vi "getReadOnly.vi"(8 "error in (no error)":errorcluster, 11 "IProperty in":refnum<class "IProperty.lvclass">) -> (0 "error out":errorcluster, 2 "Read Only?":bool, 3 "IProperty out":refnum<class "IProperty.lvclass">, 5 "Read Only?":string)   [LabVIEW 2022 SP3, in "openDAQ.lvlib" / "IBaseObject.lvlib" / "IProperty.lvlib" / "IProperty.lvclass"]
uses:
  <instrlib>/openDAQ/Public/Classes/IProperty/IProperty.lvclass
  C:/Program Files (x86)/National Instruments/LabVIEW 2022/instr.lib/openDAQ/Public/Classes/IBaseObject/IBaseObject.lvclass
  <instrlib>/openDAQ/Public/Classes/IBaseObject/IBaseObject.lvclass/IBaseObject.ctl
  <instrlib>/openDAQ/Public/Classes/IBaseObject/Accessor/Read reference.vi
  <instrlib>/openDAQ/Binaries/Windows/x86/copendaq32.dll
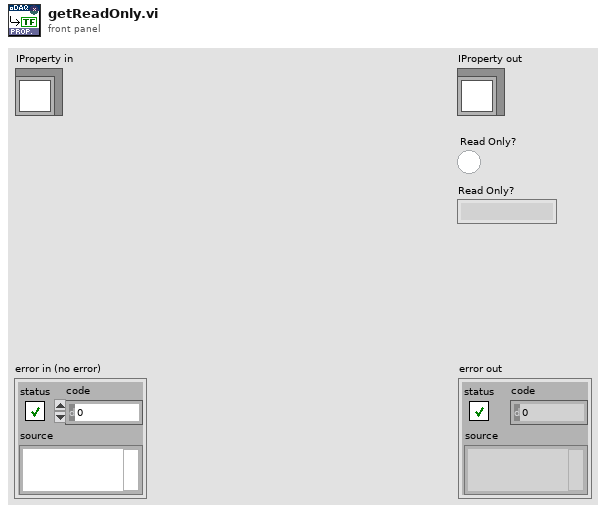
[diagram p1: front panel]
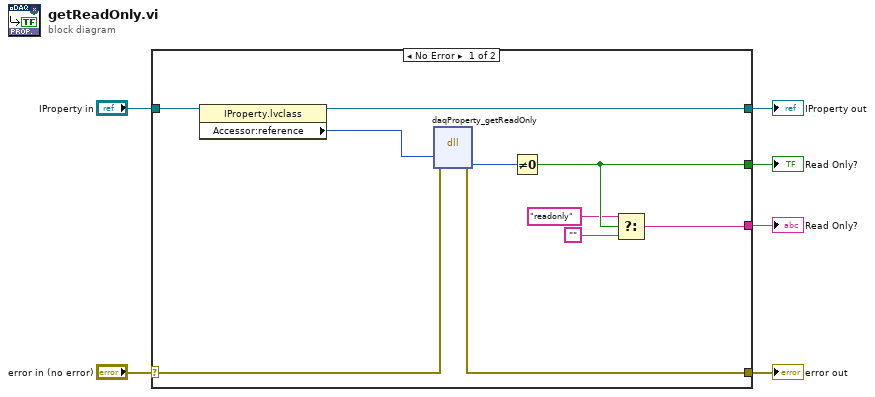
[diagram p0: block diagram]
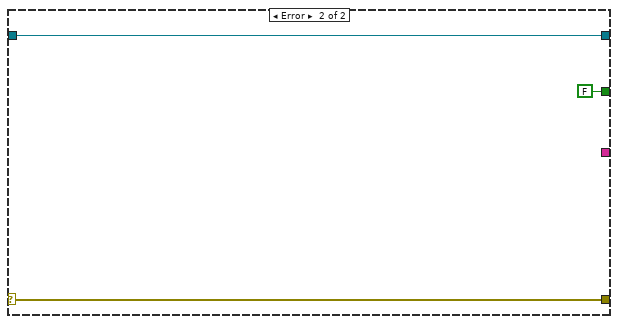
[diagram p2: hidden frame]
diagram:
  n1 = case shown="No Error" "error in (no error)" {
    selector: "error in (no error)" -> [w11 w19]
    tunnel: [w12 w19] -> w5
    tunnel: [w15 w18] -> w3
    tunnel: "IProperty in" -> [w16 w18]
    tunnel: [w10 FALSE] -> w2
    tunnel: [w7 _] -> w1
    frame No Error {
      n2 = property class="IProperty.lvclass"(reference=w16) -> (reference out=w15:refnum<class "IProperty.lvclass">, "Accessor:reference"=w14:i64)  [unwired: 1 in, 1 out]
      n3 = dll-call lib="C:/Program Files (x86)/National Instruments/LabVIEW 2022/instr.lib/openDAQ/Binaries/Windows/x86/copendaq*.*" fn="daqProperty_getReadOnly"(error in=w11, "property"=w14) -> (error out=w12:errorcluster, "readOnly"=w13:i64)  [unwired: 5 in, 1 out]
      n4 = Not Equal To 0?(x=w13) -> (x != 0?=w10:bool)
      n5 = Select(t="readonly", s=w10, f="") -> (s? t:f=w7:string)
    }
    frame Error {
    }
  }
  "error out" <- w5
  "IProperty out" <- w3
  "Read Only?" <- w2
  "Read Only?" <- w1
